vi "Load Dut.vi"(8 "error in (no error)":errorcluster, 9 "iNVMemOption":i32, 10 "USER_BIN_FILE":string, 11 "_hResourceContext":u32) -> (0 "error out":errorcluster, 1 "function return":bool, 2 "USER_BIN_FILE out":string, 3 "_hResourceContext out":u32)   [LabVIEW 2013, in "QCAWLAN_DLL.lvlib"]
doc: "QCA_DLL_Export bool LoadDut(HANDLE _hResourceContext, char* USER_BIN_FILE, int iNVMemOption);"
uses:
  QCAWLAN_DLL.lvlib
  QCAWLAN_DLL.dll
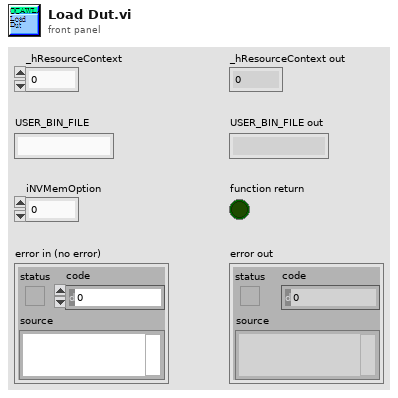
[diagram p1: front panel]
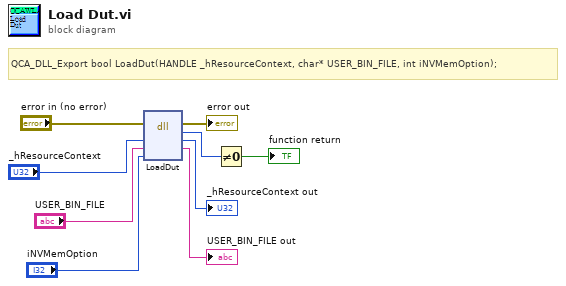
[diagram p0: block diagram]
diagram:
  # "QCA_DLL_Export bool LoadDut(HANDLE _hResourceContext, char* USER_BIN_FILE, int iNVMemOption);"
  n1 = dll-call lib="C:/Connectivity Client - MIMO/PlugIn/QCAWLAN_DLL.*" fn="LoadDut"(error in="error in (no error)", "_hResourceContext"="_hResourceContext", "USER_BIN_FILE"="USER_BIN_FILE", "iNVMemOption"="iNVMemOption") -> (error out=→"error out":errorcluster, w8:u8, "_hResourceContext"=→"_hResourceContext out":u32, "USER_BIN_FILE"=→"USER_BIN_FILE out":string)  [unwired: 3 in, 1 out]
  n2 = Not Equal To 0?(x=w8) -> (x != 0?=→"function return":bool)
